vi "optimise_lags.vi"(0 "TrajectoryDL091126GenericVoxel in":refnum<class "TrajectoryDL091126GenericVoxel.lvclass">, 1 "x command in":dbl[unit][](array[numeric]), 2 "y command in":dbl[unit][](array[numeric]), 3 "z command in":dbl[unit][](array[numeric]), 5 "x feedback in":dbl[unit][](array[numeric]), 7 "y feedback in":dbl[unit][](array[numeric]), 9 "z feedback in":dbl[unit][](array[numeric]), 11 "error in (no error)":errorcluster) -> (4 "TrajectoryDL091126GenericVoxel out":refnum<class "TrajectoryDL091126GenericVoxel.lvclass">, 15 "error out":errorcluster)   [LabVIEW 2010, in "TrajectoryDL091126GenericVoxel.lvclass"]
uses:
  TrajectoryDL091126GenericVoxel.lvclass
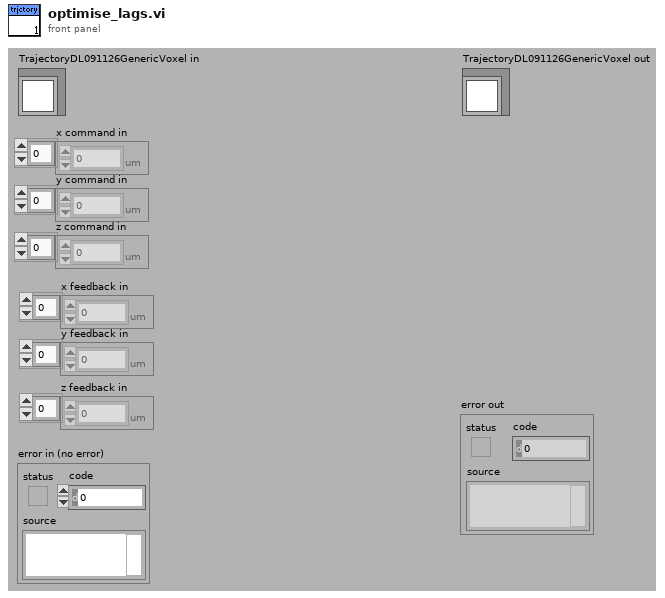
[diagram p1: front panel]
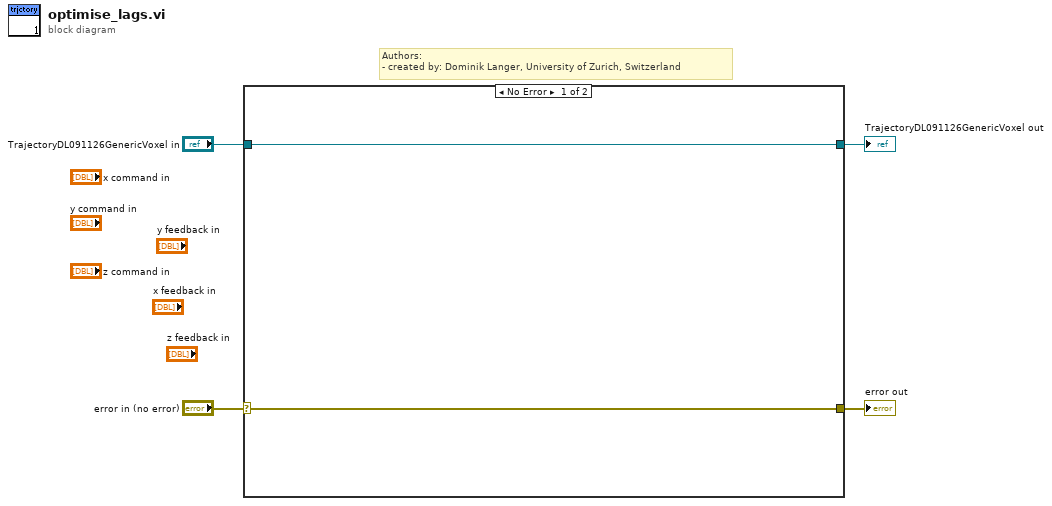
[diagram p0: block diagram]
diagram:
  # "Authors: \n- created by: Dominik Langer, University of Zurich, Switzerland"
  n1 = case shown="No Error" "error in (no error)" {
    selector: "error in (no error)" -> [w5 w8]
    tunnel: [w5 w8] -> w3
    tunnel: [w6 w7] -> w1
    tunnel: "TrajectoryDL091126GenericVoxel in" -> [w6 w7]
    frame No Error {
    }
    frame Error {
    }
  }
  "error out" <- w3
  "TrajectoryDL091126GenericVoxel out" <- w1
